vi "ejercicio 6.vi"() -> ()   [LabVIEW 2015]
panel:
  in  "Calve":string
  out "Mensaje":string
  out "Alarma":bool
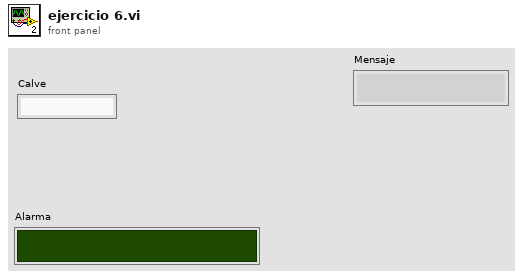
[diagram p1: front panel]
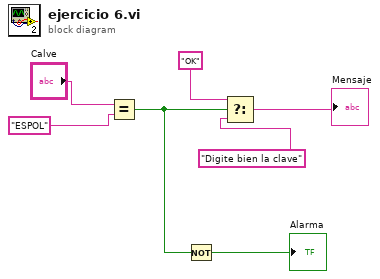
[diagram p0: block diagram]
diagram:
  n1 = Equal?(x="Calve", y="ESPOL") -> (x = y?=w3:bool)
  n2 = Not(x=w3) -> (.not. x?=→"Alarma":bool)
  n3 = Select(t="OK", s=w3, f="Digite bien la clave") -> (s? t:f=→"Mensaje":string)
